vi "Teleop.vi"(10 "Match Info":T1={"Autonomous Elapsed Seconds"=0.0, "TeleOp Elapsed Seconds"=0.0, "Disabled Elapsed Seconds"=0.0, "Visited Autonomous"=FALSE, "Visited TeleOp"=FALSE, "Visited Disabled"=FALSE, "Autonomous Settings"={"Autonomous Style"=enum."Independent", "VI Refnum"=refnum}}, 11 "Call Context":T2) -> ()   [LabVIEW 2015]
doc: "This VI is called for each TeleOp packet received from the DS where the robot is not disabled. It is often used to read from the joysticks and update I/O or to update setpoints for timed control loops. It should complete and return within 20 milliseconds or it may miss DS packets."
uses:
  <vilib>/Rock Robotics/WPI/DriverStation/WPI_DriverStationDerivedRobotMode.ctl
  <vilib>/Rock Robotics/WPI/DriverStation/WPI_DriverStationMatch Info.ctl
  <vilib>/Rock Robotics/WPI/Utilities/WPI_GetSetVariantRefNum.vi
  Robot Global Data.vi
  <vilib>/Rock Robotics/WPI/Solenoid/Deprecated/WPI_SolenoidSetBool.vi
  <vilib>/Rock Robotics/Network Tables/NT Write Boolean.vi
panel:
  in  "Multicolumn Listbox":i32(listbox)
  out "Arm Angle":dbl
  out "Voltage":dbl
  in  "LED":bool
  in  "Reset Gyro":bool
  out "Angle":dbl
  out "Shooter Speed":dbl
  out "Vision In Range":bool
  out "Vision Tracking Enabled":bool
  out "Vision Turning Value":dbl
  out "Motor Values":dbl[](array[numeric])
  # ".038\n.18\n0\n.14"
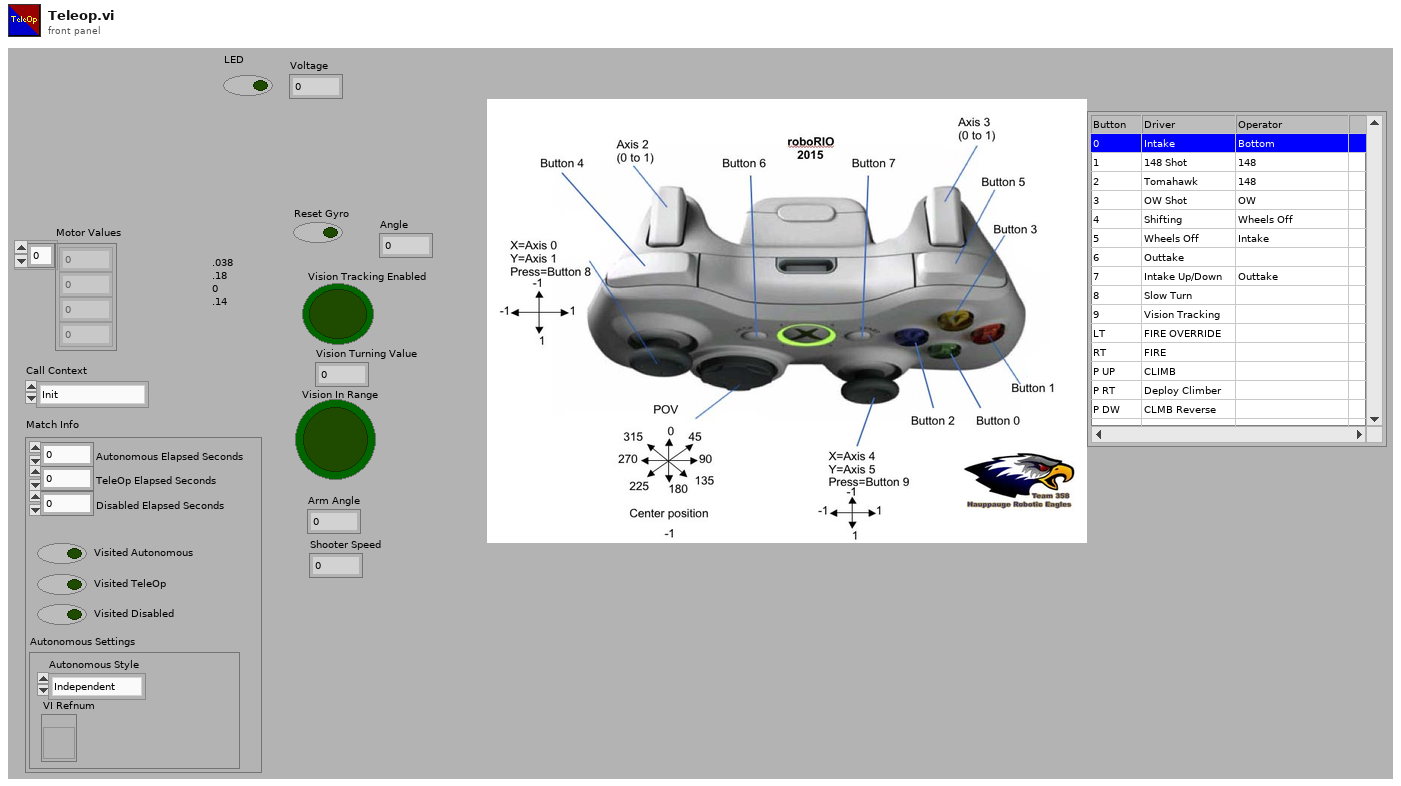
[diagram p1: front panel]
types:
  T1 = typedef "WPI_DriverStationMatch Info.ctl" = cluster{"Autonomous Elapsed Seconds":dbl, "TeleOp Elapsed Seconds":dbl, "Disabled Elapsed Seconds":dbl, "Visited Autonomous":bool, "Visited TeleOp":bool, "Visited Disabled":bool, "Autonomous Settings":cluster{"Autonomous Style":enum16{"Iterative", "Independent"}, "VI Refnum":refnum<vi>}}
  T2 = typedef "WPI_DriverStationDerivedRobotMode.ctl" = enum16{"Init", "Execute", "Stop"}
  T3 = typedef "WPI_GyroDevRef.ctl" = cluster{"DevStatus":errorcluster, "Analog Channel":T4, "Offset":dbl, "Gain (VoltsPerDegree/Second)":dbl, "Gyro Type":enum16{"Analog", "XRS450"}, "Handle":i32, "SPI Bus":T5, "Device Found":bool, "Sample Rate":dbl, "Calibrate On Open":bool}
  T4 = typedef "FPGA_AIChannel.ctl" = enum8{"AI 0", "AI 1", "AI 2", "AI 3", "AI MXP 0", "AI MXP 1", "AI MXP 2", "AI MXP 3", "Invalid"}
  T5 = typedef "spi_bus.ctl" = enum16{"SPI On-Board, CS0", "SPI On-Board, CS1", "SPI On-Board, CS2", "SPI On-Board, CS3", "SPI MXP", "Invalid"}
  T6 = typedef "WPI_AnalogChannelDevRef.ctl" = cluster{"DevStatus":errorcluster, "Analog Channel":T4}
  T7 = typedef "WPI_SolenoidDevRef.ctl" = cluster{"DevStatus":errorcluster, "Pneumatics Control Module":u8, "Forward Solenoid Channel":T8, "Reverse Solenoid Channel":T8}
  T8 = typedef "WPI_SolenoidChannel.ctl" = enum8{"Solenoid 0", "Solenoid 1", "Solenoid 2", "Solenoid 3", "Solenoid 4", "Solenoid 5", "Solenoid 6", "Solenoid 7", "Invalid"}
  T9 = typedef "WPI_MotorControlDeviceRef.ctl" = cluster{"DeviceStatus":errorcluster, "Type":T10, "PWM":cluster{"PWM Channel":T11, "DeadBand":T12}, "CAN":cluster{"Device Number":u8, "Control Mode":T13, "Semaphore":T14, "Max Vout":dbl, "TalonSRX Control Mode":T15}, "Invert":bool}
  T10 = typedef "WPI_MotorControlType.ctl" = enum16{"PWM", "CAN", "CANTalonSRX"}
  T11 = typedef "FPGA_DIOPWMChannel.ctl" = enum8{"PWM 0", "PWM 1", "PWM 2", "PWM 3", "PWM 4", "PWM 5", "PWM 6", "PWM 7", "PWM 8", "PWM 9", "PWM MXP 0", "PWM MXP 1", "PWM MXP 2", "PWM MXP 3", "PWM MXP 4", "PWM MXP 5", "PWM MXP 6", "PWM MXP 7", "PWM MXP 8", "PWM MXP 9", "Invalid"}
  T12 = typedef "WPI_PWMDeadband.ctl" = cluster{"Name":string, "maxPositivePwm":i32, "minPositivePwm":i32, "centerPwm":i32, "maxNegativePwm":i32, "minNegativePwm":i32, "angularRange":u16}
  T13 = typedef "WPI_CANJaguar_ControlMode.ctl" = enum8{"Percent VBus", "Current", "Speed", "Position", "Voltage"}
  T14 = typedef "Semaphore RefNum" = refnum<k1>
  T15 = typedef "WPI_CANTalonSRX_APIControlMode.ctl" = enum8{"Percent VBus", "Speed", "Position", "Slave", "Unchanged / Invalid", "Voltage Compensation", "Current", "Motion Profile"}
  T16 = typedef "WPI_JoystickDevRef.ctl" = cluster{"Device":T17}
  T17 = typedef "WPI_JoystickDeviceEnum.ctl" = enum16{"USB 0", "USB 1", "USB 2", "USB 3", "USB 4", "USB 5"}
  T18 = cluster{"POVs[0]":i16, "POVs[1]":i16, "POVs[2]":i16, "POVs[3]":i16, "POVs[4]":i16, "POVs[5]":i16, "POVs[6]":i16, "POVs[7]":i16, "POVs[8]":i16}
  T19 = cluster{"Axes[0]":dbl, "Axes[1]":dbl, "Axes[2]":dbl, "Axes[3]":dbl, "Axes[4]":dbl, "Axes[5]":dbl, "Axes[6]":dbl, "Axes[7]":dbl, "Axes[8]":dbl}
  T20 = cluster{"Buttons[0]":bool, "Buttons[1]":bool, "Buttons[2]":bool, "Buttons[3]":bool, "Buttons[4]":bool, "Buttons[5]":bool, "Buttons[6]":bool, "Buttons[7]":bool, "Buttons[8]":bool}
  T21 = typedef "WPI_RobotDriveDevRef.ctl" = cluster{"DevStatus":errorcluster, "Motors[]":T9[], "Square Inputs":bool, "Max Output":dbl}
  T22 = cluster{"Arm Angle":cluster{"D4":dbl, "Fender":dbl, "Low Goal":dbl, "Bottom":dbl}, "Wheel Speed":cluster{"D4":dbl, "Fender":dbl, "Low Goal":dbl, "Intake":dbl}}
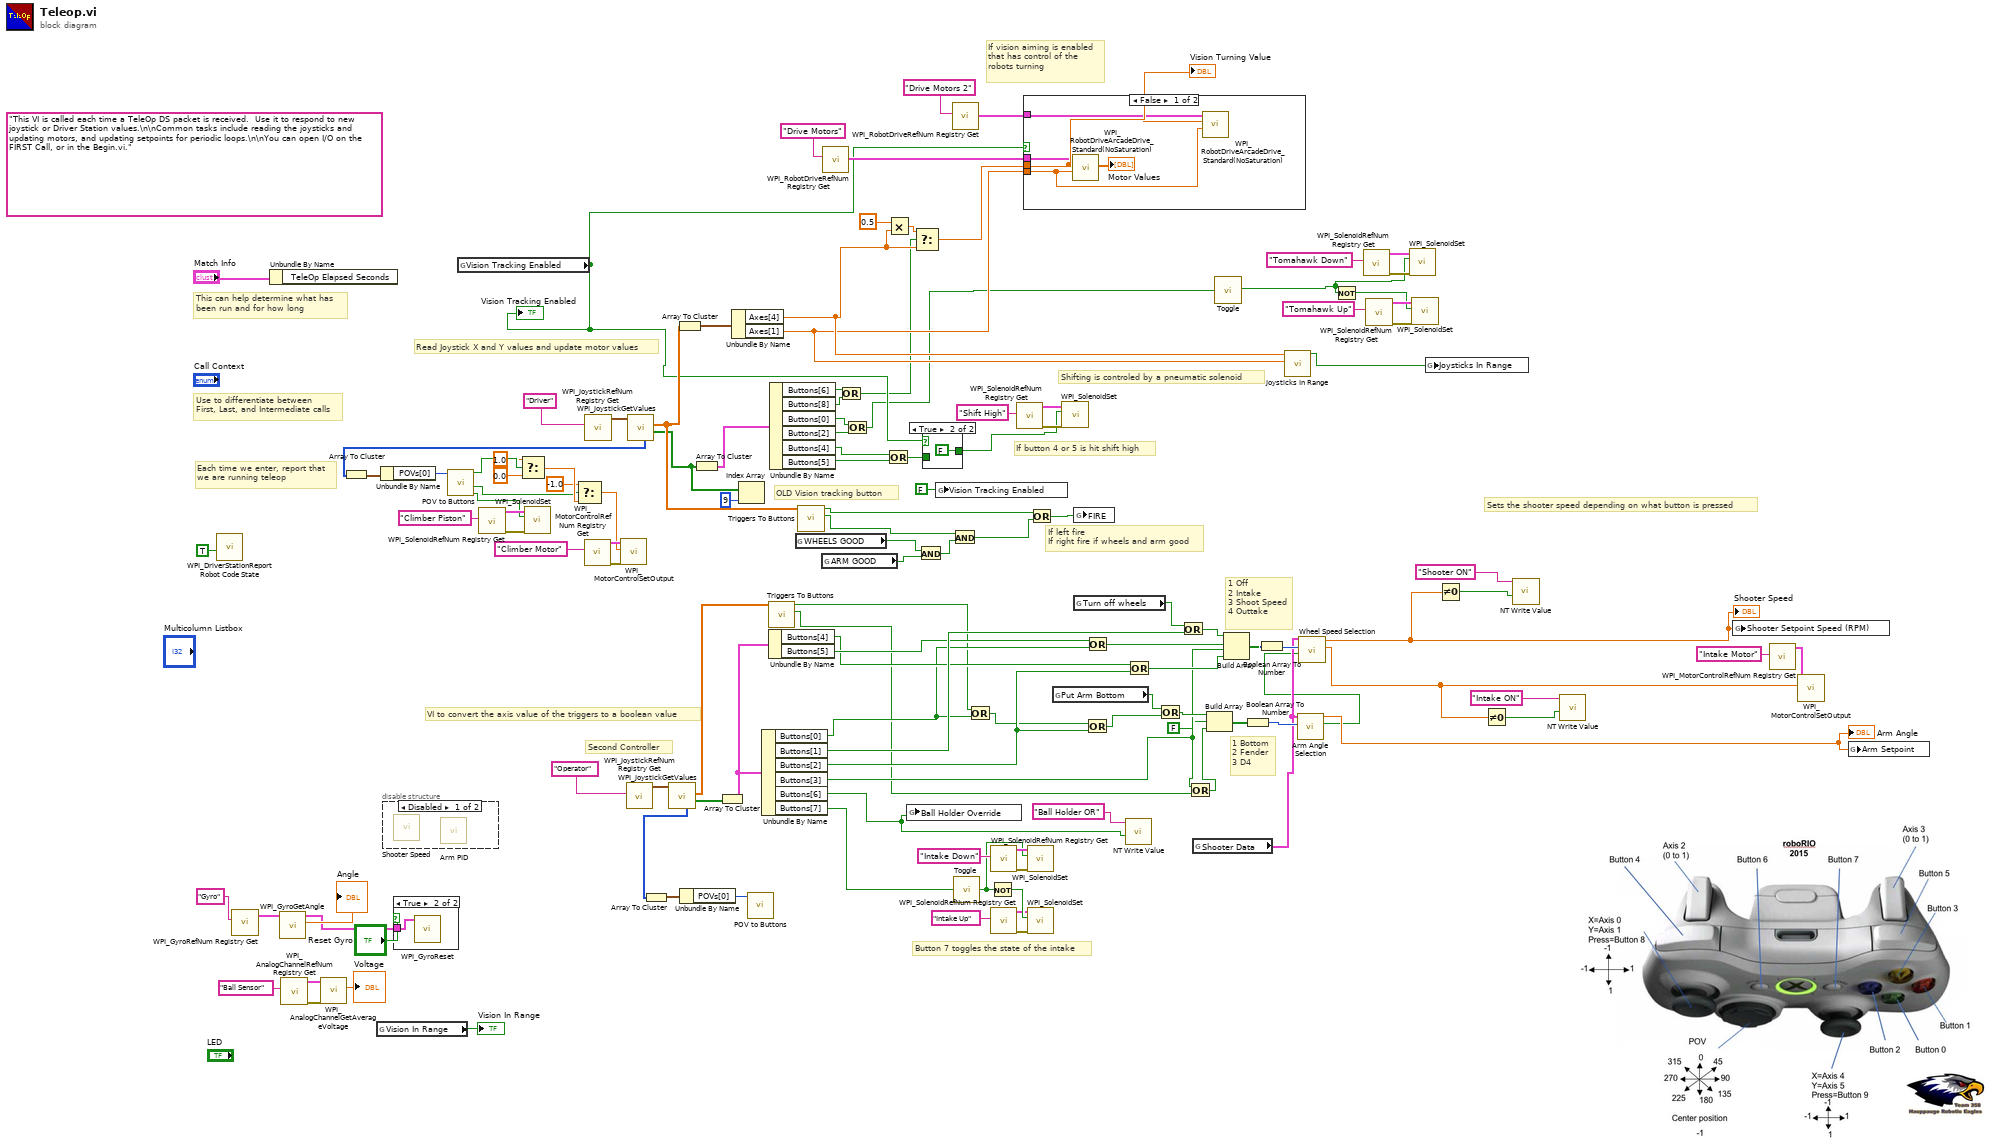
[diagram p0: block diagram]
diagram:
  (unwired) "This VI is called each time a TeleOp DS packet is received.  Use it to respond to new joystick or Driver Station values.\n\nCommon tasks include reading the joysticks and updating motors, and updating setpoints for periodic loops.\n\nYou can open I/O on the FIRST Call, or in the Begin.vi."
  # "OLD Vision tracking button"
  # "1 Off\n2 Intake\n3 Shoot Speed\n4 Outtake"
  # "1 Bottom\n2 Fender\n3 D4"
  # "If vision aiming is enabled that has control of the robots turning"
  # "VI to convert the axis value of the triggers to a boolean value"
  # "Second Controller"
  # "Button 7 toggles the state of the intake"
  # "Sets the shooter speed depending on what button is pressed"
  # "If left fire\nIf right fire if wheels and arm good"
  # "Shifting is controled by a pneumatic solenoid"
  # "If button 4 or 5 is hit shift high"
  # "Each time we enter, report that\nwe are running teleop"
  # "Use to differentiate between\nFirst, Last, and Intermediate calls"
  # "This can help determine what has\nbeen run and for how long"
  # "Read Joystick X and Y values and update motor values"
  n1 = call <vilib>:"WPI_DriverStationReport Robot Code State.vi"("TeleOp"=TRUE ("Autonomous")) -> ()  [unwired: 10 in, 1 out]
  n2 = call <vilib>:"WPI_GyroRefNum Registry Get.vi"("refnum name"="Gyro") -> ("GyroDevRef"=w87:T3)  [unwired: 9 in, 1 out]
  n3 = Unbundle By Name("Match Info") -> ()  [unwired: 1 out]
  n4 = call <vilib>:"WPI_GyroGetAngle.vi"("GyroDevRef"=w87) -> ("Angle"=→"Angle":dbl, "GyroDevRef"=w85:T3)  [unwired: 6 in, 3 out]
  n5 = call <vilib>:"WPI_AnalogChannelRefNum Registry Get.vi"("refnum name"="Ball Sensor") -> ("error out"=w83:errorcluster, "AIDeviceRef"=w82:T6)  [unwired: 9 in]
  n6 = call <vilib>:"WPI_AnalogChannelGetAverageVoltage.vi"("error in (no error)"=w83, "AIDeviceRef"=w82) -> ("Voltage"=→"Voltage":dbl)  [unwired: 7 in, 2 out]
  n7 = global read "Robot Global Data.vi" "Vision In Range"() -> (→"Vision In Range":bool)
  n8 = disable-structure shown="Disabled" {
    frame Disabled {
      n9 = call "Shooter Speed.vi"() -> ()  [unwired: 2 in]
      n10 = call "Arm PID.vi"() -> ()  [unwired: 12 in]
    }
    frame Enabled {
    }
  }
  n11 = case shown="True" "Reset Gyro" {
    tunnel: w85 -> [_ w129]
    frame False {
    }
    frame True {
      n12 = call <vilib>:"WPI_GyroReset.vi"("GyroDevRef"=w129) -> ()  [unwired: 9 in, 2 out]
    }
  }
  n13 = global read "Robot Global Data.vi" "Vision Tracking Enabled"() -> (w74:bool)
  "Vision Tracking Enabled" <- w74
  n14 = call <vilib>:"WPI_SolenoidRefNum Registry Get.vi"("refnum name"="Climber Piston") -> ("error out"=w59:errorcluster, "SolenoidDevRef"=w60:T7)  [unwired: 9 in]
  n15 = call <vilib>:"WPI_MotorControlRefNum Registry Get.vi"("refnum name"="Climber Motor") -> ("error out"=w58:errorcluster, "MotorControlDevRef"=w57:T9)  [unwired: 9 in]
  n16 = call <vilib>:"WPI_JoystickRefNum Registry Get.vi"("refnum name"="Driver") -> ("JoystickDevRef"=w124:T16)  [unwired: 1 in, 9 out]
  n17 = call <vilib>:"WPI_JoystickRefNum Registry Get.vi"("refnum name"="Operator") -> ("JoystickDevRef"=w104:T16)  [unwired: 1 in, 9 out]
  n18 = call <vilib>:"WPI_JoystickGetValues.vi"("JoystickDevRef"=w124) -> ("Buttons"=w38:bool[], "Axes"=w99:dbl[], "POVs"=w62:i16[])  [unwired: 6 in, 2 out]
  n19 = Array To Cluster(array=w62) -> (cluster=w63:T18)
  n20 = Unbundle By Name(w63) -> ("POVs[0]"=w64:i16)
  n21 = call "POV to Buttons.vi"("POV Input"=w64) -> ("Right"=w40:bool, "Down"=w53:bool, "Up"=w52:bool)  [unwired: 7 in, 1 out]
  n22 = Select(t=1.0, s=w52, f=0.0) -> (s? t:f=w55:dbl)
  n23 = call-poly <vilib>:"WPI_SolenoidSet.vi"("error in (no error)"=w59, "Value"=w40, "SolenoidDevRef"=w60) -> ()  [unwired: 7 in, 2 out]
  n24 = Select(t=-1.0, s=w53, f=w55) -> (s? t:f=w54:dbl)
  n25 = call <vilib>:"WPI_MotorControlSetOutput.vi"("error in (no error)"=w58, "Output"=w54, "MotorControlDevRef"=w57) -> ()  [unwired: 6 in, 3 out]
  n26 = call <vilib>:"WPI_JoystickGetValues.vi"("JoystickDevRef"=w104) -> ("Buttons"=w102:bool[], "Axes"=w100:dbl[], "POVs"=w101:i16[])  [unwired: 6 in, 2 out]
  n27 = Array To Cluster(array=w101) -> (cluster=w108:T18)
  n28 = Array To Cluster(array=w99) -> (cluster=w122:T19)
  n29 = Unbundle By Name(w108) -> ("POVs[0]"=w107:i16)
  n30 = Array To Cluster(array=w38) -> (cluster=w39:T20)
  n31 = Array To Cluster(array=w102) -> (cluster=w44:T20)
  n32 = Unbundle By Name(w122) -> ("Axes[4]"=w48:dbl, "Axes[1]"=w47:dbl)
  n33 = Index Array(array=w38, index=9) -> ()  [unwired: 1 out]
  n34 = call "POV to Buttons.vi"("POV Input"=w107) -> ()  [unwired: 7 in, 4 out]
  n35 = Unbundle By Name(w44) -> ("Buttons[0]"=w20:bool, "Buttons[1]"=w26:bool, "Buttons[2]"=w23:bool, "Buttons[3]"=w17:bool, "Buttons[6]"=w14:bool, "Buttons[7]"=w13:bool)
  n36 = call "Triggers To Buttons.vi"("Axes"=w100) -> ("Right"=w15:bool, "Left"=w18:bool)  [unwired: 9 in]
  n37 = Unbundle By Name(w44) -> ("Buttons[4]"=w21:bool, "Buttons[5]"=w24:bool)
  n38 = Unbundle By Name(w39) -> ("Buttons[6]"=w10:bool, "Buttons[8]"=w9:bool, "Buttons[0]"=w4:bool, "Buttons[2]"=w3:bool, "Buttons[4]"=w7:bool, "Buttons[5]"=w6:bool)
  n39 = global read "Robot Global Data.vi" "WHEELS GOOD"() -> (w68:bool)
  n40 = call "Triggers To Buttons.vi"("Axes"=w99) -> ("Right"=w66:bool, "Left"=w70:bool)  [unwired: 9 in]
  n41 = global read "Robot Global Data.vi" "ARM GOOD"() -> (w69:bool)
  n42 = call <vilib>:"WPI_RobotDriveRefNum Registry Get.vi"("refnum name"="Drive Motors") -> ("RobotDriveDevRef"=w126:T21)  [unwired: 1 in, 9 out]
  n43 = Or(x=w10, y=w9) -> (x .or. y?=w5:bool)
  n44 = Or(x=w4, y=w3) -> (x .or. y?=w2:bool)
  n45 = Or(x=w7, y=w6) -> (x .or. y?=w11:bool)
  n46 = Multiply(x=0.5, y=w48) -> (x*y=w72:dbl)
  n47 = global write "Robot Global Data.vi" "Ball Holder Override"(w14) -> ()
  n48 = Select(t=w72, s=w5, f=w48) -> (s? t:f=w73:dbl)
  "Vision Turning Value" <- w73
  n49 = And(x=w68, y=w69) -> (x .and. y?=w67:bool)
  n50 = case shown="True" w74 {
    tunnel: [w130 FALSE] -> w97
    tunnel: w11 -> [w130 _]
    frame False {
    }
    frame True {
    }
  }
  n51 = global write "Robot Global Data.vi" "Vision Tracking Enabled"(FALSE ("Vision Tracking Enabled")) -> ()
  n52 = And(x=w66, y=w67) -> (x .and. y?=w65:bool)
  n53 = call <vilib>:"WPI_RobotDriveRefNum Registry Get.vi"("refnum name"="Drive Motors 2") -> ("RobotDriveDevRef"=w110:T21)  [unwired: 1 in, 9 out]
  n54 = call "Toggle.vi"("Input"=w13) -> ("Output"=w111:bool)
  n55 = Or(x=w18, y=w20) -> (x .or. y?=w19:bool)
  n56 = Not(x=w111) -> (.not. x?=w118:bool)
  n57 = call <vilib>:"WPI_SolenoidRefNum Registry Get.vi"("refnum name"="Intake Down") -> ("error out"=w112:errorcluster, "SolenoidDevRef"=w113:T7)  [unwired: 9 in]
  n58 = call <vilib>:"WPI_SolenoidRefNum Registry Get.vi"("refnum name"="Intake Up") -> ("error out"=w117:errorcluster, "SolenoidDevRef"=w116:T7)  [unwired: 9 in]
  n59 = call <vilib>:"WPI_SolenoidRefNum Registry Get.vi"("refnum name"="Shift High") -> ("error out"=w121:errorcluster, "SolenoidDevRef"=w120:T7)  [unwired: 9 in]
  n60 = case shown="False" w74 {
    tunnel: w126 -> [w136 _]
    tunnel: w110 -> [w134 _]
    tunnel: w47 -> [w133 _]
    tunnel: w73 -> [w132 _]
    frame False {
      n61 = call <vilib>:"WPI_RobotDriveArcadeDrive_Standard(NoSaturation).vi"("Y axis value"=w133, "X axis value"=w132, "RobotDriveDevRef"=w136) -> ("Motor Values"=→"Motor Values":dbl[])  [unwired: 1 in, 7 out]
      n62 = call <vilib>:"WPI_RobotDriveArcadeDrive_Standard(NoSaturation).vi"("Y axis value"=w133, "X axis value"=w132, "RobotDriveDevRef"=w134) -> ()  [unwired: 1 in, 8 out]
    }
    frame True {
    }
  }
  n63 = call-poly <vilib>:"WPI_SolenoidSet.vi"("error in (no error)"=w112, "Value"=w111, "SolenoidDevRef"=w113) -> ()  [unwired: 7 in, 2 out]
  n64 = call-poly <vilib>:"WPI_SolenoidSet.vi"("error in (no error)"=w117, "Value"=w118, "SolenoidDevRef"=w116) -> ()  [unwired: 7 in, 2 out]
  n65 = Or(x=w70, y=w65) -> (x .or. y?=w75:bool)
  n66 = global read "Robot Global Data.vi" "Put Arm Bottom"() -> (w42:bool)
  n67 = call-poly <vilib>:"WPI_SolenoidSet.vi"("error in (no error)"=w121, "Value"=w97, "SolenoidDevRef"=w120) -> ()  [unwired: 7 in, 2 out]
  n68 = global write "Robot Global Data.vi" "FIRE"(w75) -> ()
  n69 = global read "Robot Global Data.vi" "Turn off wheels"() -> (w29:bool)
  n70 = Or(x=w19, y=w23) -> (x .or. y?=w27:bool)
  n71 = Or(x=w24, y=w20) -> (x .or. y?=w25:bool)
  n72 = call-poly <vilib>:"NT Write Value.vi"("Boolean"=w14, "Name"="Ball Holder OR") -> ()  [unwired: 9 in, 1 out]
  n73 = Or(x=w21, y=w23) -> (x .or. y?=w22:bool)
  n74 = Or(x=w42, y=w27) -> (x .or. y?=w41:bool)
  n75 = Or(x=w29, y=w26) -> (x .or. y?=w28:bool)
  n76 = Or(x=w17, y=w15) -> (x .or. y?=w16:bool)
  n77 = global read "Robot Global Data.vi" "Shooter Data"() -> (w76:T22)
  n78 = Build Array(w41, FALSE ("element"), w16) -> (w45:bool[])
  n79 = call "Toggle.vi"("Input"=w2) -> ("Output"=w90:bool)
  n80 = Build Array(w28, w25, w17, w22) -> (w1:bool[])
  n81 = Boolean Array To Number(Boolean array=w45) -> (number=w79:u32)
  n82 = Boolean Array To Number(Boolean array=w1) -> (number=w78:u32)
  n83 = call "Joysticks In Range.vi"("y"=w47, "x"=w48) -> ("x .and. y?"=w46:bool)  [unwired: 9 in]
  n84 = call "Arm Angle Selection.vi"("Numeric Control"=w79, "Shooter Data"=w76) -> ("D4 Angle"=w43:bool, "Arm Setpoint"=w77:dbl)  [unwired: 8 in]
  "Arm Angle" <- w77
  n85 = call "Wheel Speed Selection.vi"("D4?"=w43, "Numeric Control"=w78, "Shooter Data"=w76) -> ("Intake Speed"=w31:dbl, "Shooter Speed"=w36:dbl)  [unwired: 6 in, 1 out]
  "Shooter Speed" <- w36
  n86 = Not(x=w90) -> (.not. x?=w91:bool)
  n87 = call <vilib>:"WPI_SolenoidRefNum Registry Get.vi"("refnum name"="Tomahawk Down") -> ("error out"=w96:errorcluster, "SolenoidDevRef"=w89:T7)  [unwired: 9 in]
  n88 = call <vilib>:"WPI_SolenoidRefNum Registry Get.vi"("refnum name"="Tomahawk Up") -> ("error out"=w92:errorcluster, "SolenoidDevRef"=w93:T7)  [unwired: 9 in]
  n89 = call-poly <vilib>:"WPI_SolenoidSet.vi"("error in (no error)"=w96, "Value"=w90, "SolenoidDevRef"=w89) -> ()  [unwired: 7 in, 2 out]
  n90 = call-poly <vilib>:"WPI_SolenoidSet.vi"("error in (no error)"=w92, "Value"=w91, "SolenoidDevRef"=w93) -> ()  [unwired: 7 in, 2 out]
  n91 = global write "Robot Global Data.vi" "Joysticks In Range"(w46) -> ()
  n92 = Not Equal To 0?(x=w36) -> (x != 0?=w35:bool)
  n93 = Not Equal To 0?(x=w31) -> (x != 0?=w32:bool)
  n94 = call-poly <vilib>:"NT Write Value.vi"("Boolean"=w35, "Name"="Shooter ON") -> ()  [unwired: 9 in, 1 out]
  n95 = call-poly <vilib>:"NT Write Value.vi"("Boolean"=w32, "Name"="Intake ON") -> ()  [unwired: 9 in, 1 out]
  n96 = global write "Robot Global Data.vi" "Shooter Setpoint Speed (RPM)"(w36) -> ()
  n97 = call <vilib>:"WPI_MotorControlRefNum Registry Get.vi"("refnum name"="Intake Motor") -> ("MotorControlDevRef"=w105:T9)  [unwired: 9 in, 1 out]
  n98 = call <vilib>:"WPI_MotorControlSetOutput.vi"("Output"=w31, "MotorControlDevRef"=w105) -> ()  [unwired: 7 in, 3 out]
  n99 = global write "Robot Global Data.vi" "Arm Setpoint"(w77) -> ()
